vi "FlushSamples.vi"(8 "error in (no error)":errorcluster, 11 "FitterBase in":refnum<class "FitterBase.lvclass">) -> (0 "error out":errorcluster, 3 "FitterBase out":refnum<class "FitterBase.lvclass">)   [LabVIEW 2018, in "AnalysisPlugins.lvlib" / "FitterBase.lvclass"]
uses:
  FitterBase.lvclass
  C:/projects/ICDAS/NistPluggableModules/Analysis/AnalysisPlugins/AnalysisPluginBaseClass/AnalysisPluginsBase.lvclass
  AnalysisPluginBaseClass/Typedefs/SampleDataInput.ctl
  AnalysisPluginBaseClass/AnalysisPluginsBase.lvclass/AnalysisPluginsBase.ctl
  AnalysisPluginBaseClass/Accessors/Read SampleDataQueName.vi
  AnalysisPluginBaseClass/AnalysisPluginsBase.lvclass
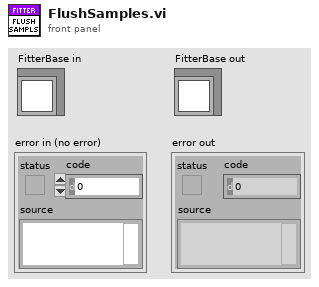
[diagram p1: front panel]
types:
  T1 = typedef "AnalysisPlugins.lvlib/AnalysisPluginsBase.lvclass/SampleDataInput.ctl" = waveform(dbl)[]
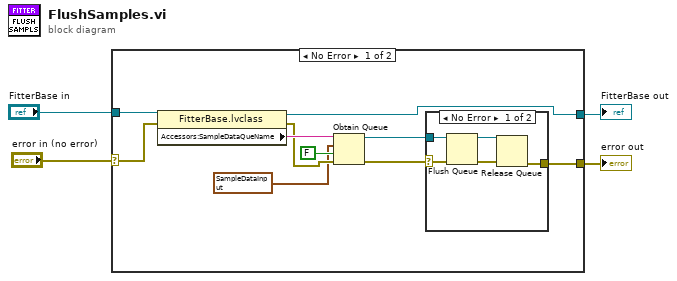
[diagram p0: block diagram]
diagram:
  n1 = case shown="No Error" "error in (no error)" {
    selector: "error in (no error)" -> [w13 w21]
    tunnel: "FitterBase in" -> [w14 w20]
    tunnel: [w6 w20] -> w2
    tunnel: [w5 w21] -> w1
    frame No Error {
      n2 = property class="FitterBase.lvclass"(reference=w14, error in=w13) -> (reference out=w6:refnum<class "FitterBase.lvclass">, error out=w11:errorcluster, "Accessors:SampleDataQueName"=w12:string)
      n3 = Obtain Queue(name (unnamed)=w12, element data type=T1 [{"t0"=timestamp(0 s since 1904-01-01), "dt"=1.0, "Y"=[]}] ("clSampleDataArray"), create if not found? (T)=FALSE, error in (no error)=w11) -> (queue out=w8:refnum<queue>, error out=w7:errorcluster)  [unwired: 1 in, 1 out]
      n4 = case shown="No Error" w7 {
        selector: w7 -> [w19 _]
        tunnel: w8 -> [w18 _]
        tunnel: [w15 _] -> w5
        frame No Error {
          n5 = Flush Queue(queue=w18, error in (no error)=w19) -> (queue out=w16:refnum<queue>, error out=w17:errorcluster)  [unwired: 1 out]
          n6 = Release Queue(queue=w16, error in (no error)=w17) -> (error out=w15:errorcluster)  [unwired: 1 in, 2 out]
        }
        frame Error {
          # "Do not pass the error"
        }
      }
    }
    frame Error {
    }
  }
  "error out" <- w1
  "FitterBase out" <- w2
